vi "Actor Core.vi"(8 "error in":errorcluster, 11 "ActorAutoRegistrationView In":refnum<class "ActorAutoRegistrationView.lvclass">) -> (0 "error out":errorcluster, 3 "Actor out":refnum<class "Actor.lvclass">)   [LabVIEW 2015, in "TestViewables.lvlib" / "ActorAutoRegistrationView.lvclass"]
doc: "(<B>Filename</B>: Actor Framework.lvlib:Actor.lvclass:Actor Core.vi)\n\nReceives messages to the actor, reacts to them, and initiates any error handling that may shut the actor down.\n\nDescendant classes may override this VI to append parallel tasks for the actor to complete while it handles messages. Overrides use the Call Parent Method node.\n\n<License>\nCopyright © 2017 Composed Systems, LLC | All rights reserved\nwww.composed.io\n\nAuthor: Ethan Stern <ethan.stern@composed.io>\n\nThis software is provided \"AS IS\" WITHOUT WARRANTIES, either express or implied, AND IS FOR EDUCATIONAL PURPOSES ONLY.\n</License>"
uses:
  ActorAutoRegistrationView.lvclass
  <vilib>/ActorFramework/Actor/Actor.lvclass
  <vilib>/ActorFramework/Actor/Actor.lvclass/Actor.ctl
  <vilib>/ActorFramework/Message Enqueuer/Message Enqueuer.lvclass/Message Enqueuer.ctl
  Framework/AutoRegistration/ActorAutoRegistration/ActorAutoRegistration.lvclass/ActorAutoRegistration.ctl
  <vilib>/ActorFramework/Message Enqueuer/Init from Existing Queue.vi
  Framework/AutoRegistration/AutoRegistration/Register for Panel Events.vi
  Framework/IViewable/IViewable/IViewable.lvclass
  <vilib>/ActorFramework/Message Enqueuer/Message Enqueuer.lvclass
  Framework/AutoRegistration/ActorAutoRegistration/ActorAutoRegistration.lvclass
panel:
  in  "Latch When Released":bool
  in  "Latch Until Released":bool
  in  "Switch Until Released":bool
  in  "Switch When Released":bool
  in  "Latch When Pressed":bool
  in  "Switch When Pressed":bool
  # "An actor implementing full auto-registration"
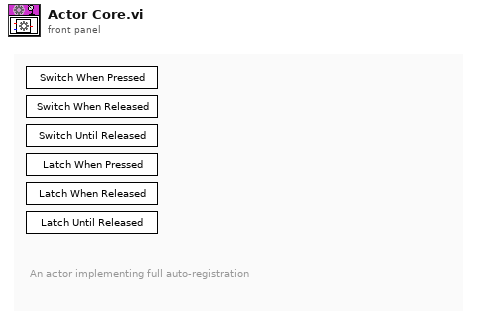
[diagram p1: front panel]
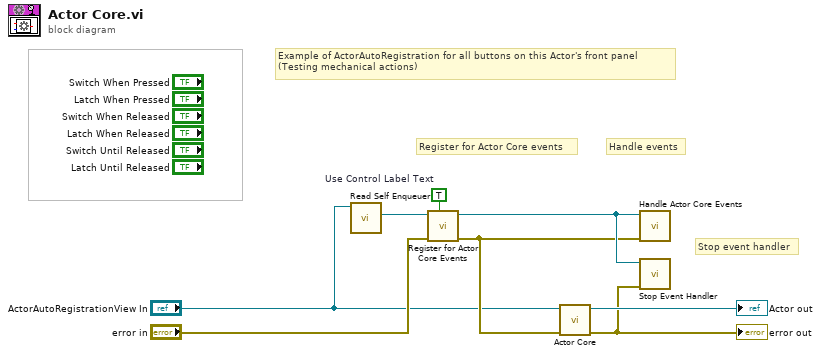
[diagram p0: block diagram]
diagram:
  w4 = TRUE  # Use Control Label Text
  # "Example of ActorAutoRegistration for all buttons on this Actor's front panel\n(Testing mechanical actions)"
  # "Stop event handler"
  # "Handle events"
  # "Register for Actor Core events"
  n1 = call <vilib>:"Read Self Enqueuer.vi"("Actor"="ActorAutoRegistrationView In") -> ("Self Enqueuer"=w7:refnum<class "Message Enqueuer.lvclass">)  [unwired: 10 in]
  n2 = call "Register for Actor Core Events.vi"("Use Label Text (F=Use Caption)"=w4, "error in (no error)"="error in", "Actor Enqueuer"=w7) -> ("error out"=w2:errorcluster, "ActorAutoRegistration Out"=w5:refnum<class "ActorAutoRegistration.lvclass">)  [unwired: 7 in]
  n3 = call-parent "Actor Core.vi"("error in"=w2, "IViewable In"="ActorAutoRegistrationView In") -> ("error out"=w6:errorcluster, "Actor out"=→"Actor out":refnum<class "Actor.lvclass">)  [unwired: 8 in]
  "error out" <- w6
  n4 = call-dynamic "Handle Actor Core Events.vi"("error in (no error)"=w2, "ActorAutoRegistration"=w5) -> ()  [unwired: 9 in, 1 out]
  n5 = call-dynamic "Stop Event Handler.vi"("error in (no error)"=w6, "ActorAutoRegistration In"=w5) -> ()  [unwired: 9 in, 1 out]
